vi "GL Command Set.vi"(5 "Command":T2=enum."Abort Motion", 7 "Text Input":string, 8 "error in (no error)":errorcluster, 9 "Value":i32, 10 "Axis":T1 items=["Axis 1", "Axis 2", "Axis 3", "Axis 4", "Axis 5", "Axis 6", "Axis 7", "Axis 8"], 11 "Galil.IGalil":refnum<k7>) -> (0 "error out":errorcluster, 1 "Response#":i32, 2 "Axis Out":T1 items=["Axis 1", "Axis 2", "Axis 3", "Axis 4", "Axis 5", "Axis 6", "Axis 7", "Axis 8"], 3 "ref out":refnum<k7>, 6 "Response: text":string)   [LabVIEW 2022 SP3]
doc: "Sets the operation mode for an axis or vector space."
uses:
  Command Menu.ctl
  GL Axis Control.ctl
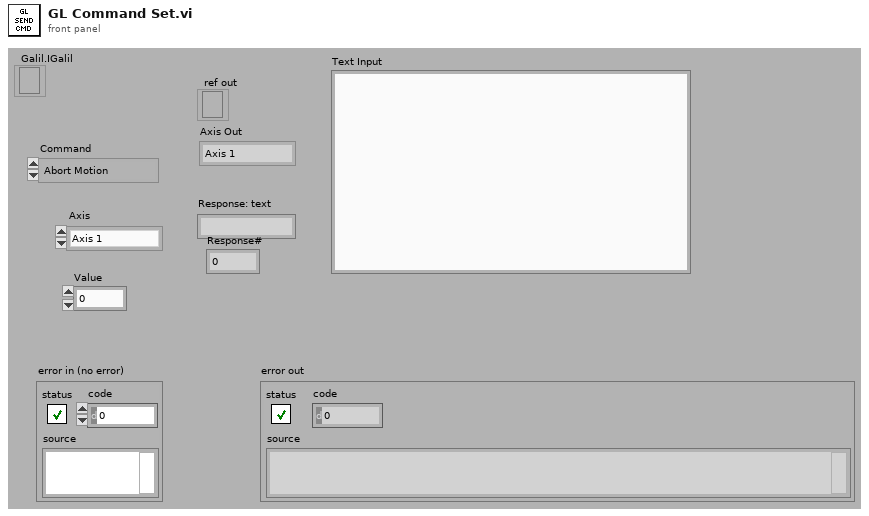
[diagram p1: front panel]
types:
  T1 = typedef "GL Axis Control.ctl" = u16
  T2 = typedef "Command Menu.ctl" = enum16{"CommandPassThrough", "Abort Motion", "Define Pos", "Velocity", "Acceleration", "Deceleration", "Position Rel", "Postion Abs", "Begin Move", "After Move", "Home", "KI", "KD", "KP", "IL", "Config I/O", "Set Bit", "Clear Bit", "Motor Off", "Moto On", "Status", "Execute", "Halt Execute", "HX Status", "Tell Velocity", "Check Motion", "BreakPoint", "Tell Position", "Current Code Line", "Tell Switches", "OC Force On", "OC Off", "Pos Soft Limit", "Rev Soft Limit"}
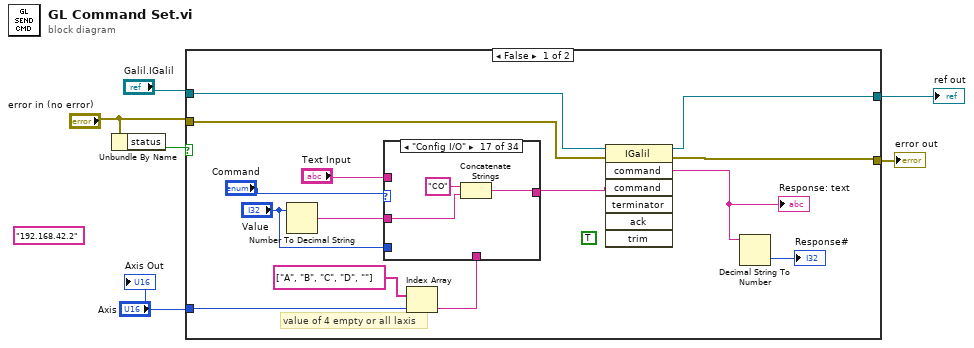
[diagram p0: block diagram]
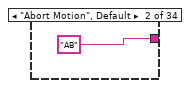
[diagram p3: hidden frame]
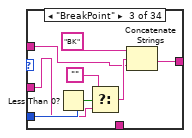
[diagram p4: hidden frame]
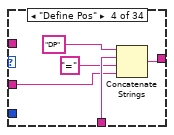
[diagram p5: hidden frame]
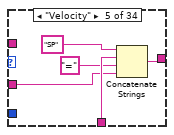
[diagram p6: hidden frame]
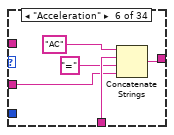
[diagram p7: hidden frame]
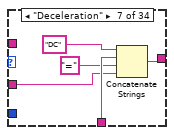
[diagram p8: hidden frame]
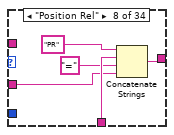
[diagram p9: hidden frame]
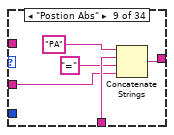
[diagram p10: hidden frame]
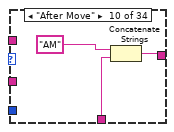
[diagram p11: hidden frame]
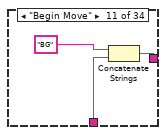
[diagram p12: hidden frame]
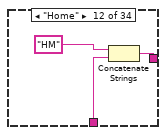
[diagram p13: hidden frame]
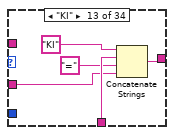
[diagram p14: hidden frame]
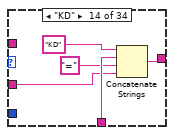
[diagram p15: hidden frame]
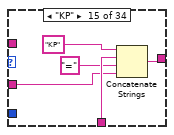
[diagram p16: hidden frame]
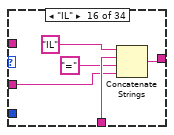
[diagram p17: hidden frame]
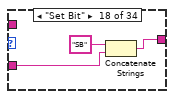
[diagram p18: hidden frame]
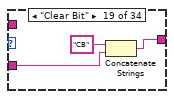
[diagram p19: hidden frame]
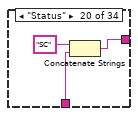
[diagram p20: hidden frame]
diagram:
  (unwired) "192.168.42.2"
  n1 = Unbundle By Name("error in (no error)") -> ("status"=w4:bool)
  n2 = case shown="False" w4 {
    tunnel: "error in (no error)" -> [w11 w153]
    tunnel: [w10 w153] -> w5
    tunnel: "Galil.IGalil" -> [w14 w152]
    tunnel: [w13 w152] -> w3
    tunnel: "Axis" -> [w7 _]
    frame False {
      (unwired) TRUE ("trim")
      # "value of 4 empty or all laxis"
      n3 = Number To Decimal String(number="Value") -> (decimal integer string=w17:string)  [unwired: 1 in]
      n4 = Index Array(array=string[] ["A", "B", "C", "D", ""], index=w7) -> (element=w18:string)
      n5 = case shown="\"Config I/O\"" "Command" {
        tunnel: [w21 "AB" w29 w31 w36 w41 w46 w51 w56 w62 w64 w67 w70 w75 w80 w85 w90 w94 w97 w100 w103 w109 w112 w114 w118 w120 w124 w127 "OCA=0" "OCA=_TPA,0" w134 w140 w146 w151] -> w12
        tunnel: w18 -> [_ _ _ w34 w39 w44 w49 w54 w59 w61 w65 w68 w73 w78 w83 w88 _ _ _ w99 _ _ w111 w115 w117 w121 w123 w126 _ _ _ _ w144 w149]
        tunnel: w17 -> [_ _ w26 w32 w37 w42 w47 w52 w57 _ _ _ w71 w76 w81 w86 w91 w93 w96 _ w102 _ _ _ _ _ _ _ _ _ w133 w139 w143 w148]
        tunnel: "Text Input" -> [w21 _ w23 _ _ _ _ _ _ _ _ _ _ _ _ _ _ _ _ _ w105 w108 _ _ _ _ _ _ _ _ _ _ _ _]
        tunnel: "Value" -> [_ _ w28 _ _ _ _ _ _ _ _ _ _ _ _ _ _ _ _ _ _ _ _ _ _ _ _ _ _ _ w131 _ _ _]
        frame "CommandPassThrough" {
        }
        frame "Abort Motion", Default {
        }
        frame "BreakPoint" {
          n6 = Less Than 0?(x=w28) -> (x < 0?=w27:bool)
          n7 = Select(t="", s=w27, f=w26) -> (s? t:f=w24:string)
          n8 = Concatenate Strings("BK", w24, w23) -> (w29:string)
        }
        frame "Define Pos" {
          n9 = Concatenate Strings("DP", w34, "=" ("string"), w32) -> (w31:string)
        }
        frame "Velocity" {
          n10 = Concatenate Strings("SP", w39, "=" ("string"), w37) -> (w36:string)
        }
        frame "Acceleration" {
          n11 = Concatenate Strings("AC", w44, "=" ("string"), w42) -> (w41:string)
        }
        frame "Deceleration" {
          n12 = Concatenate Strings("DC", w49, "=" ("string"), w47) -> (w46:string)
        }
        frame "Position Rel" {
          n13 = Concatenate Strings("PR", w54, "=" ("string"), w52) -> (w51:string)
        }
        frame "Postion Abs" {
          n14 = Concatenate Strings("PA", w59, "=" ("string"), w57) -> (w56:string)
        }
        frame "After Move" {
          n15 = Concatenate Strings("AM", w61) -> (w62:string)
        }
        frame "Begin Move" {
          n16 = Concatenate Strings("BG", w65) -> (w64:string)
        }
        frame "Home" {
          n17 = Concatenate Strings("HM", w68) -> (w67:string)
        }
        frame "KI" {
          n18 = Concatenate Strings("KI", w73, "=" ("string"), w71) -> (w70:string)
        }
        frame "KD" {
          n19 = Concatenate Strings("KD", w78, "=" ("string"), w76) -> (w75:string)
        }
        frame "KP" {
          n20 = Concatenate Strings("KP", w83, "=" ("string"), w81) -> (w80:string)
        }
        frame "IL" {
          n21 = Concatenate Strings("IL", w88, "=" ("string"), w86) -> (w85:string)
        }
        frame "Config I/O" {
          n22 = Concatenate Strings("CO", w91) -> (w90:string)
        }
        frame "Set Bit" {
          n23 = Concatenate Strings("SB", w93) -> (w94:string)
        }
        frame "Clear Bit" {
          n24 = Concatenate Strings("CB", w96) -> (w97:string)
        }
        frame "Status" {
          n25 = Concatenate Strings("SC", w99) -> (w100:string)
        }
        frame "Execute" {
          n26 = Concatenate Strings("XQ ", w105, "," ("string"), w102) -> (w103:string)
        }
        frame "Current Code Line" {
          n27 = Concatenate Strings("LS ", w108, ",0" ("string")) -> (w109:string)
        }
        frame "Tell Velocity" {
          n28 = Concatenate Strings("TV", w111) -> (w112:string)
        }
        frame "Check Motion" {
          n29 = Concatenate Strings("MG_BG" ("command"), w115) -> (w114:string)
        }
        frame "Motor Off" {
          n30 = Concatenate Strings("MO" ("command"), w117) -> (w118:string)
        }
        frame "Moto On" {
          n31 = Concatenate Strings("SH" ("command"), w121) -> (w120:string)
        }
        frame "Tell Position" {
          n32 = Concatenate Strings("TP", w123) -> (w124:string)
        }
        frame "Tell Switches" {
          n33 = Concatenate Strings("TS", w126) -> (w127:string)
        }
        frame "OC Off" {
        }
        frame "OC Force On" {
        }
        frame "Halt Execute" {
          n34 = case shown="0, Default" w131 {
            tunnel: [w137 w138] -> w134
            tunnel: w133 -> [w136 _]
            tunnel: "HX" ("string") -> [w135 w138]
            frame 0, Default {
              n35 = Concatenate Strings(w135, w136) -> (w137:string)
            }
            frame -1 {
            }
          }
        }
        frame "HX Status" {
          n36 = Concatenate Strings("MG _HX" ("string"), w139) -> (w140:string)
        }
        frame "Pos Soft Limit" {
          n37 = Concatenate Strings("FL " ("string"), w144, "= " ("string"), w143) -> (w146:string)
        }
        frame "Rev Soft Limit" {
          n38 = Concatenate Strings("BL " ("string"), w149, "= " ("string"), w148) -> (w151:string)
        }
      }
      n39 = invoke class="IGalil" method="command"(reference=w14, error in=w11, "command"=w12) -> (reference out=w13:refnum<k7>, error out=w10:errorcluster, "command"=w9:string)  [unwired: 4 in, 4 out]
      "Response: text" <- w9
      n40 = Decimal String To Number(string=w9) -> (number=→"Response#":i32)  [unwired: 2 in, 1 out]
    }
    frame True {
    }
  }
  "error out" <- w5
  "ref out" <- w3
  "Axis Out" <- "Axis"
